vi "toXml.vi"(8 "error in (no error)":errorcluster, 11 "RampEvent in":refnum<class "RampEvent.lvclass">) -> (0 "error out":errorcluster, 2 "scriptEventXML":refnum<class "xmlNode.lvclass">, 3 "RampEvent out":refnum<class "RampEvent.lvclass">)   [LabVIEW 2011, in "Tools.lvlib" / "Scripting.lvlib" / "RampEvent.lvclass"]
uses:
  RampEvent.lvclass
  xmlNode/xmlNode.lvclass
  DatabaseHelpers/Database Objects/Channel/Channel.lvclass
  ScriptEvent.lvclass
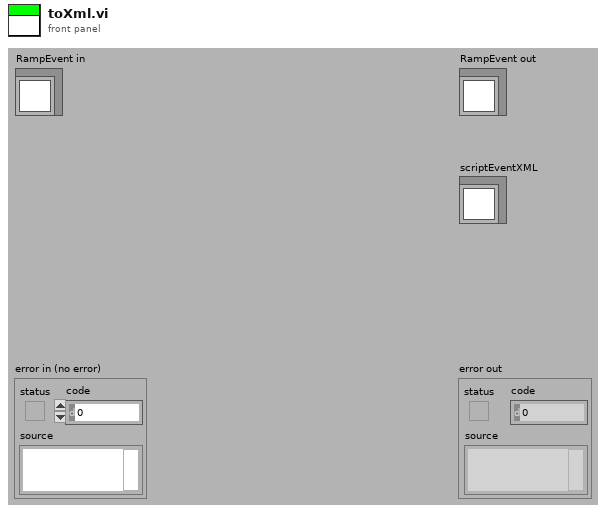
[diagram p1: front panel]
types:
  T1 = cluster{"attributeName":string, "channel_name":string}
  T2 = cluster{"attributeName":string, "channel_name":string}[]
  T3 = cluster{"parameter_name":string, "parameter_value":string, "type":enum16{"time", "time_difference", "value", "frequency", "phase", "ramp_time", "value_step", "time_step", "number_of_steps", "start_value", "end_value", "start_freq", "start_amp", "start_phase", "end_freq", "end_amp", "end_phase"}}[]
  T4 = enum16{"time", "time_difference", "value", "frequency", "phase", "ramp_time", "value_step", "time_step", "number_of_steps", "start_value", "end_value", "start_freq", "start_amp", "start_phase", "end_freq", "end_amp", "end_phase"}
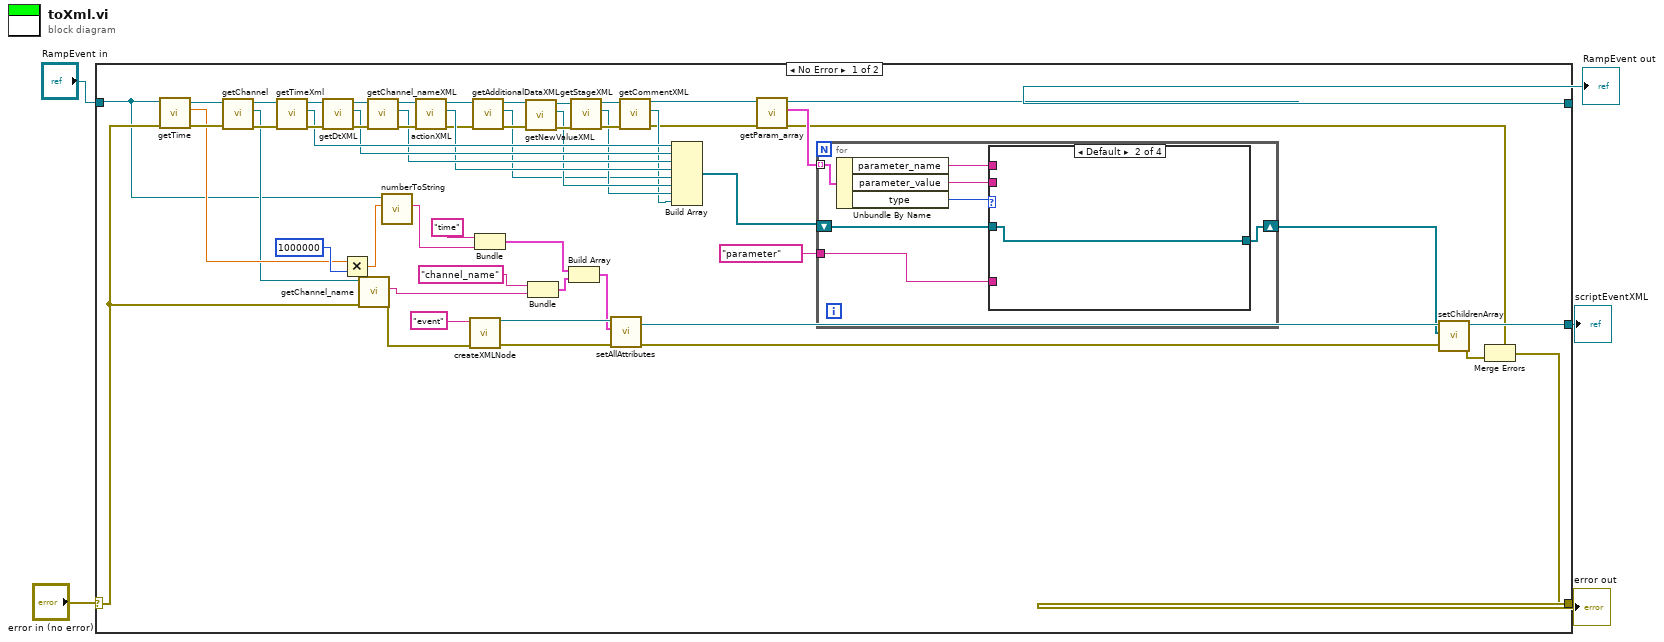
[diagram p0: block diagram]
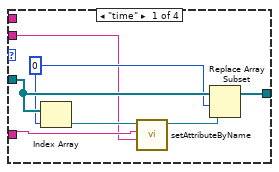
[diagram p2: hidden frame]
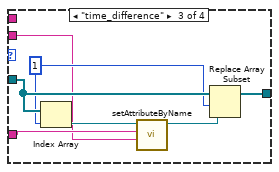
[diagram p3: hidden frame]
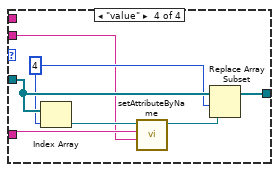
[diagram p4: hidden frame]
diagram:
  n1 = case shown="No Error" "error in (no error)" {
    selector: "error in (no error)" -> [w24 w92]
    tunnel: "RampEvent in" -> [w16 w91]
    tunnel: [w9 w91] -> w3
    tunnel: [w23 w92] -> w2
    tunnel: [w31 _] -> w1
    frame No Error {
      n2 = call "getTime.vi"("error in (no error)"=w24, "ScriptEvent.lvclass in"=w16) -> ("error out"=w29:errorcluster, "time"=w26:dbl, "ScriptEvent.lvclass out"=w27:refnum<class "RampEvent.lvclass">)  [unwired: 7 in]
      n3 = call-dynamic "getChannel.vi"("error in (no error)"=w29, "ScriptEvent.lvclass in"=w27) -> ("error out"=w30:errorcluster, "Channel.lvclass"=w25:refnum<class "Channel.lvclass">, "ScriptEvent.lvclass out"=w28:refnum<class "RampEvent.lvclass">)  [unwired: 7 in]
      n4 = call "getTimeXml.vi"("error in (no error)"=w30, "ScriptEvent in"=w28) -> ("error out"=w59:errorcluster, "timeXML"=w49:refnum<class "xmlNode.lvclass">, "ScriptEvent out"=w54:refnum<class "RampEvent.lvclass">)  [unwired: 7 in]
      n5 = call "getDtXML.vi"("error in (no error)"=w59, "ScriptEvent in"=w54) -> ("error out"=w58:errorcluster, "dtXML"=w48:refnum<class "xmlNode.lvclass">, "ScriptEvent out"=w53:refnum<class "RampEvent.lvclass">)  [unwired: 7 in]
      n6 = Multiply(x=w26, y=1000000) -> (x*y=w15:dbl)
      n7 = call "getChannel_name.vi"("error in (no error)"=w24, "Channel.lvclass in"=w25) -> ("error out"=w60:errorcluster, "channel_name"=w40:string)  [unwired: 7 in, 1 out]
      n8 = call "getChannel_nameXML.vi"("error in (no error)"=w58, "ScriptEvent in"=w53) -> ("error out"=w57:errorcluster, "channel_nameXML"=w47:refnum<class "xmlNode.lvclass">, "ScriptEvent out"=w52:refnum<class "RampEvent.lvclass">)  [unwired: 7 in]
      n9 = call "numberToString.vi"("Numeric"=w15, "ScriptEvent in"=w16) -> ("String"=w14:string)  [unwired: 7 in, 2 out]
      n10 = call "actionXML.vi"("error in (no error)"=w57, "ScriptEvent in"=w52) -> ("error out"=w20:errorcluster, "actionXml"=w46:refnum<class "xmlNode.lvclass">, "ScriptEvent out"=w22:refnum<class "RampEvent.lvclass">)  [unwired: 7 in]
      n11 = call "createXMLNode.vi"("error in (no error)"=w60, "name"="event") -> ("error out"=w35:errorcluster, "xmlNode out"=w39:refnum<class "xmlNode.lvclass">)  [unwired: 8 in]
      n12 = call-dynamic "getAdditionalDataXML.vi"("error in (no error)"=w20, "RampEvent in"=w22) -> ("error out"=w19:errorcluster, "additionalDataXML"=w18:refnum<class "xmlNode.lvclass">, "RampEvent out"=w21:refnum<class "RampEvent.lvclass">)  [unwired: 7 in]
      n13 = Bundle("attributeName"="time", "String"=w14) -> (w38:cluster{"attributeName":string, "String":string})  [unwired: 1 in]
      n14 = call-dynamic "getNewValueXML.vi"("error in (no error)"=w19, "RampEvent in"=w21) -> ("error out"=w56:errorcluster, "newValueXML"=w45:refnum<class "xmlNode.lvclass">, "RampEvent out"=w51:refnum<class "RampEvent.lvclass">)  [unwired: 7 in]
      n15 = Bundle("attributeName"="channel_name", "channel_name"=w40) -> (w37:T1)  [unwired: 1 in]
      n16 = Build Array(w38, w37) -> (w36:T2)
      n17 = call "getStageXML.vi"("error in (no error)"=w56, "ScriptEvent in"=w51) -> ("error out"=w55:errorcluster, "stageXML"=w44:refnum<class "xmlNode.lvclass">, "ScriptEvent out"=w50:refnum<class "RampEvent.lvclass">)  [unwired: 7 in]
      n18 = call-dynamic "setAllAttributes.vi"("error in (no error)"=w35, "attributes"=w36, "xmlNode in"=w39) -> ("error out"=w34:errorcluster, "xmlNode out"=w33:refnum<class "xmlNode.lvclass">)  [unwired: 7 in]
      n19 = call "getCommentXML.vi"("error in (no error)"=w55, "ScriptEvent in"=w50) -> ("error out"=w11:errorcluster, "commentXML"=w17:refnum<class "xmlNode.lvclass">, "ScriptEvent out"=w10:refnum<class "RampEvent.lvclass">)  [unwired: 7 in]
      n20 = Build Array(w49, w48, w47, w46, w18, w45, w44, w17) -> (w6:refnum<class "xmlNode.lvclass">[])
      n21 = call "getParam_array.vi"("error in (no error)"=w11, "ScriptEvent in"=w10) -> ("error out"=w8:errorcluster, "param_array"=w12:T3, "ScriptEvent out"=w9:refnum<class "RampEvent.lvclass">)  [unwired: 7 in]
      n22 = for {
        tunnel: w12 -> [w68] mode=indexing
        shift-right: [w63] -> w7
        shift-left: w6 -> [w66]
        tunnel: "parameter" -> [w62]
        n23 = Unbundle By Name(w68) -> ("parameter_name"=w65:string, "parameter_value"=w64:string, "type"=w67:T4)
        n24 = case shown="Default" w67 {
          tunnel: w66 -> [w73 w76 w81 w88]
          tunnel: w65 -> [_ _ _ _]
          tunnel: w64 -> [w69 _ w77 w84]
          tunnel: [w71 w76 w79 w86] -> w63
          tunnel: w62 -> [w70 _ w78 w85]
          frame "time" {
            w72 = 0
            n25 = Index Array(array=w73, index=w72) -> (element=w75:refnum<class "xmlNode.lvclass">)
            n26 = call-dynamic "setAttributeByName.vi"("attributeValue"=w69, "attributeName"=w70, "xmlNode in"=w75) -> ("xmlNode out"=w74:refnum<class "xmlNode.lvclass">)  [unwired: 7 in, 1 out]
            n27 = Replace Array Subset(array=w73, new element=w74, index=w72) -> (w71:refnum<class "xmlNode.lvclass">[])
          }
          frame Default {
          }
          frame "time_difference" {
            w80 = 1
            n28 = Index Array(array=w81, index=w80) -> (element=w83:refnum<class "xmlNode.lvclass">)
            n29 = call-dynamic "setAttributeByName.vi"("attributeValue"=w77, "attributeName"=w78, "xmlNode in"=w83) -> ("xmlNode out"=w82:refnum<class "xmlNode.lvclass">)  [unwired: 7 in, 1 out]
            n30 = Replace Array Subset(array=w81, new element=w82, index=w80) -> (w79:refnum<class "xmlNode.lvclass">[])
          }
          frame "value" {
            w87 = 4
            n31 = Index Array(array=w88, index=w87) -> (element=w90:refnum<class "xmlNode.lvclass">)
            n32 = call-dynamic "setAttributeByName.vi"("attributeValue"=w84, "attributeName"=w85, "xmlNode in"=w90) -> ("xmlNode out"=w89:refnum<class "xmlNode.lvclass">)  [unwired: 7 in, 1 out]
            n33 = Replace Array Subset(array=w88, new element=w89, index=w87) -> (w86:refnum<class "xmlNode.lvclass">[])
          }
        }
      }
      n34 = call-dynamic "setChildrenArray.vi"("error in (no error)"=w34, "Children"=w7, "xmlNode.lvclass in"=w33) -> ("error out"=w43:errorcluster, "xmlNode.lvclass out"=w31:refnum<class "xmlNode.lvclass">)  [unwired: 7 in]
      n35 = Merge Errors(w8, w43) -> (w23:errorcluster)
    }
    frame Error {
    }
  }
  "error out" <- w2
  "RampEvent out" <- w3
  "scriptEventXML" <- w1
